vi "RT Loop - Host Messaging.vi"(0 "Message Queue":refnum<queue>) -> ()   [LabVIEW 2017]
uses:
  Support/Message Queue/Message Cluster.ctl
  Globals/Host/Global - Configuration Options.vi
  Globals/RT/Globals - RT Stream.vi
  Support/Message Queue/Message Queue.lvlib
  <resource>/objmgr/ni.dex.rc
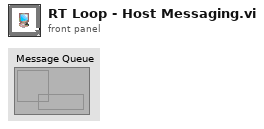
[diagram p1: front panel]
types:
  T1 = enum16{"UI Connection Polling", "Listen For UI Commands"}
  T2 = typedef "Message Queue.lvlib/Message Cluster.ctl" = cluster{"Message":string, "Message Data":variant}
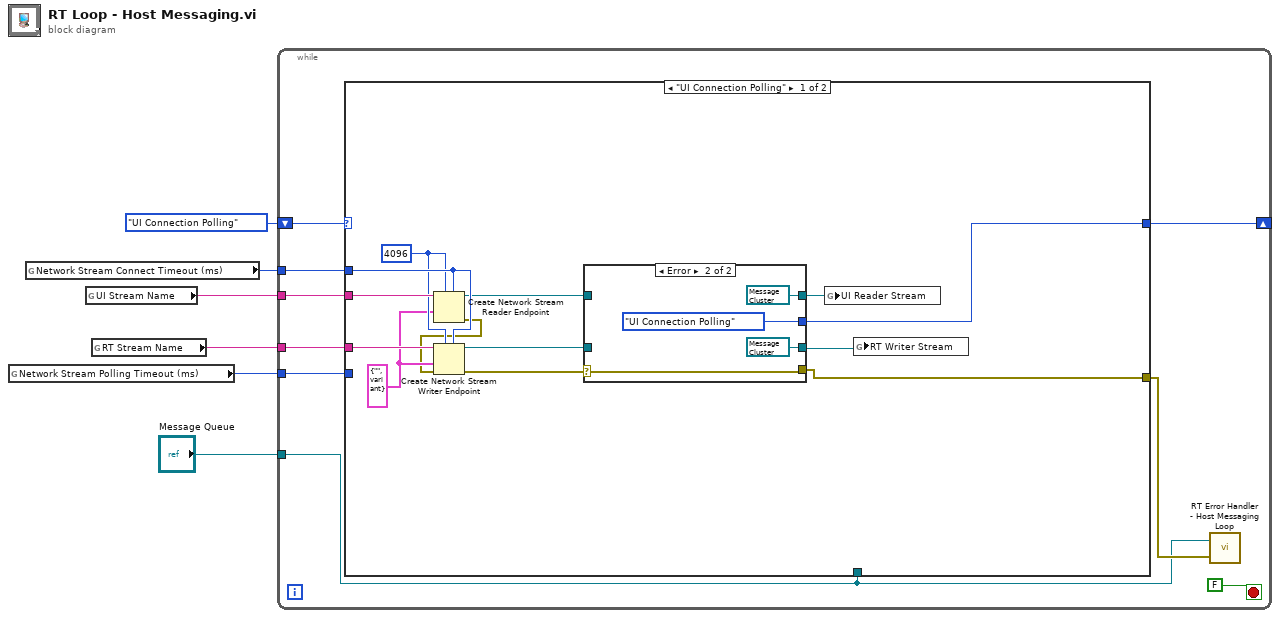
[diagram p0: block diagram]
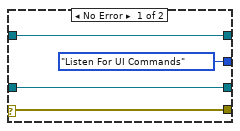
[diagram p2: hidden frame]
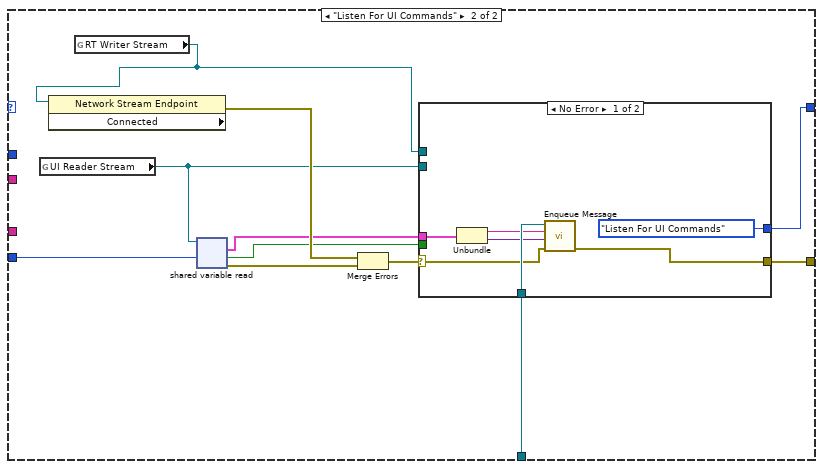
[diagram p3: hidden frame]
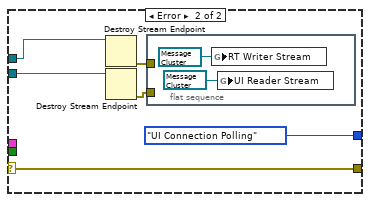
[diagram p4: hidden frame]
diagram:
  n1 = global read "Global - Configuration Options.vi" "Network Stream Polling Timeout (ms)"() -> (w1:i32)
  n2 = global read "Global - Configuration Options.vi" "Network Stream Connect Timeout (ms)"() -> (w2:i32)
  n3 = global read "Global - Configuration Options.vi" "UI Stream Name"() -> (w4:string)
  n4 = global read "Global - Configuration Options.vi" "RT Stream Name"() -> (w3:string)
  n5 = while {
    tunnel: "Message Queue" -> [w8]
    tunnel: w4 -> [w14]
    tunnel: w3 -> [w13]
    tunnel: w2 -> [w12]
    shift-right: [w11] -> _
    shift-left: T1."UI Connection Polling" -> [w15]
    tunnel: w1 -> [w10]
    stop <- FALSE ("stop") stop-if-true
    n6 = case shown="\"UI Connection Polling\"" w15 {
      tunnel: w14 -> [w28 _]
      tunnel: w13 -> [w27 _]
      tunnel: w12 -> [w26 _]
      tunnel: [w19 w41] -> w11
      tunnel: w10 -> [_ w47]
      tunnel: w8 -> [_ w40]
      tunnel: [w18 w39] -> w9
      frame "UI Connection Polling" {
        w24 = T2 {"Message"="", "Message Data"=variant} ("Message Cluster")
        w25 = 4096 ("reader buffer size")
        n7 = Create Network Stream Reader Endpoint(5:w26, 7:w25, 9:w24, 11:w28) -> (0:w23:errorcluster, 3:w20:refnum<k21>)  [unwired: 3 in]
        n8 = Create Network Stream Writer Endpoint(5:w26, 7:w25, 8:w23, 9:w24, 11:w27) -> (0:w22:errorcluster, 3:w21:refnum<k21>)  [unwired: 2 in]
        n9 = case shown="Error" w22 {
          selector: w22 -> [w29 w33]
          tunnel: w21 -> [w32 _]
          tunnel: w20 -> [w31 _]
          tunnel: [w32 refnum<k21> refnum ("RT Stream Name")] -> w16
          tunnel: [w31 refnum<k21> refnum ("UI Stream Name")] -> w17
          tunnel: [T1."Listen For UI Commands" T1."UI Connection Polling"] -> w19
          tunnel: [w29 w33] -> w18
          frame No Error {
          }
          frame Error {
          }
        }
        n10 = global write "Globals - RT Stream.vi" "UI Reader Stream"(w17) -> ()
        n11 = global write "Globals - RT Stream.vi" "RT Writer Stream"(w16) -> ()
      }
      frame "Listen For UI Commands" {
        n12 = global read "Globals - RT Stream.vi" "UI Reader Stream"() -> (w37:refnum<k21>)
        n13 = global read "Globals - RT Stream.vi" "RT Writer Stream"() -> (w38:refnum<k21>)
        n14 = property class="Network Stream Endpoint" props=["Connected"](reference=w38) -> (error out=w45:errorcluster)  [unwired: 1 in, 2 out]
        n15 = shared-variable-read(w37, w47) -> (w44:errorcluster, w43:bool, w42:T2)  [unwired: 1 in, 1 out]
        n16 = Merge Errors(w45, w44) -> (w46:errorcluster)
        n17 = case shown="No Error" w46 {
          selector: w46 -> [w50 w55]
          tunnel: w43 -> [_ _]
          tunnel: w42 -> [w53 _]
          tunnel: w37 -> [_ w59]
          tunnel: w38 -> [_ w60]
          tunnel: [T1."Listen For UI Commands" T1."UI Connection Polling"] -> w41
          tunnel: w40 -> [w54 _]
          tunnel: [w49 w55] -> w39
          frame No Error {
            n18 = Unbundle(w53) -> ("Message"=w52:string, "Message Data"=w51:variant)
            n19 = call "Enqueue Message.vi"("error in (no error)"=w50, "Message Data"=w51, "Message"=w52, "Message Queue"=w54) -> ("error out"=w49:errorcluster)  [unwired: 6 in, 1 out]
          }
          frame Error {
            n20 = Destroy Stream Endpoint(11:w60) -> (0:w58:errorcluster)  [unwired: 1 in]
            n21 = Destroy Stream Endpoint(11:w59) -> (0:w57:errorcluster)  [unwired: 1 in]
            n22 = flat-sequence {
              tunnel: w58 -> [_]
              tunnel: w57 -> [_]
              frame #0 {
                n23 = global write "Globals - RT Stream.vi" "RT Writer Stream"(refnum<k21> refnum ("UI Command Stream")) -> ()
                n24 = global write "Globals - RT Stream.vi" "UI Reader Stream"(refnum<k21> refnum ("RT Message Stream")) -> ()
              }
            }
          }
        }
      }
    }
    n25 = call "RT Error Handler - Host Messaging Loop.vi"("Error In"=w9, "Message Queue"=w8) -> ()  [unwired: 1 in]
  }
